vi "UI_sendComplexMessage.vi"(5 "Notif T/O":i32=250, 6 "notifier":refnum<notifier>, 7 "Wait for Response":bool, 8 "error in (no error)":errorcluster, 9 "Payload":variant, 10 "Command":string, 11 "Queue Bus":T1) -> (0 "error out":errorcluster, 1 "payload":variant, 3 "Queue Bus OUT":T1)   [LabVIEW 2020]
uses:
  Typedefs/queueBus.ctl
  Typedefs/communicationData.ctl
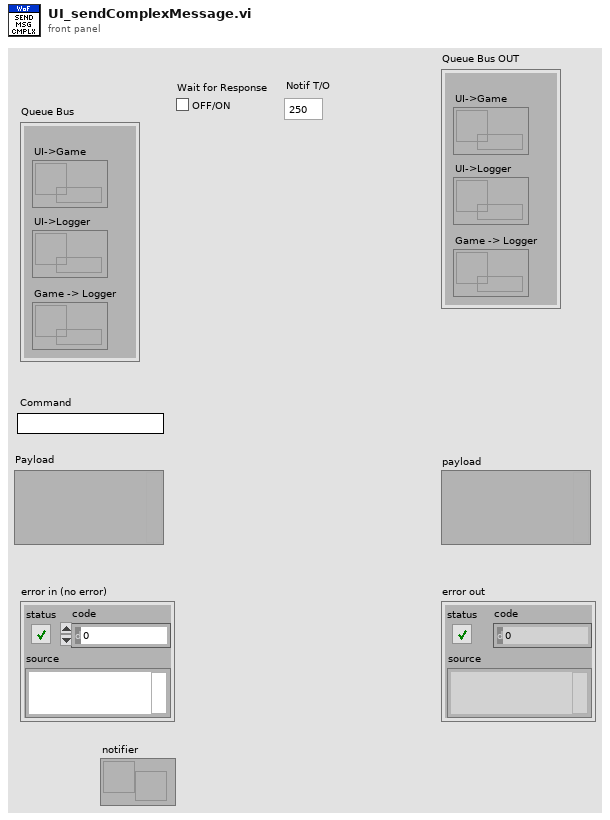
[diagram p1: front panel]
types:
  T1 = typedef "queueBus.ctl" = cluster{"UI->Game":refnum<queue>, "UI->Logger":refnum<queue>, "Game -> Logger":refnum<queue>}
  T2 = typedef "communicationData.ctl" = cluster{"command":string, "payload":variant, "response":variant}
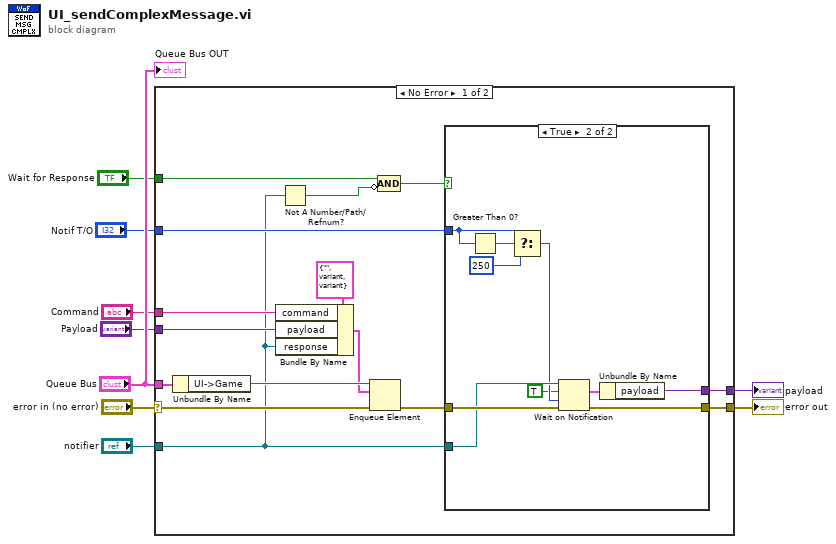
[diagram p0: block diagram]
diagram:
  n1 = case shown="No Error" "error in (no error)" {
    selector: "error in (no error)" -> [w22 w36]
    tunnel: [w15 w36] -> w7
    tunnel: "notifier" -> [w12 _]
    tunnel: "Queue Bus" -> [w24 _]
    tunnel: "Payload" -> [w19 _]
    tunnel: "Command" -> [w20 _]
    tunnel: "Wait for Response" -> [w17 _]
    tunnel: "Notif T/O" -> [w14 _]
    tunnel: [w13 _] -> w1
    frame No Error {
      n2 = Unbundle By Name(w24) -> ("UI->Game"=w23:refnum<queue>)
      n3 = Bundle By Name(cluster=T2 {"command"="", "payload"=variant, "response"=variant} ("communication"), "command"=w20, "payload"=w19, "response"=w12) -> (w18:T2)
      n4 = Not A Number/Path/Refnum?(number/path/refnum=w12) -> (NaN/Path/Refnum?=w10:bool)
      n5 = Enqueue Element(queue=w23, element=w18, error in (no error)=w22) -> (error out=w16:errorcluster)  [unwired: 1 in, 2 out]
      n6 = Compound Arithmetic op=AND(w17, invert w10) -> (w11:bool)
      n7 = case shown="True" w11 {
        tunnel: w16 -> [w25 w35]
        tunnel: [w25 w34] -> w15
        tunnel: w12 -> [_ w33]
        tunnel: w14 -> [_ w31]
        tunnel: [_ w26] -> w13
        frame False {
        }
        frame True {
          n8 = Greater Than 0?(x=w31) -> (x > 0?=w32:bool)
          n9 = Select(t=w31, s=w32, f=250) -> (s? t:f=w29:i32)
          n10 = Wait on Notification(notifier=w33, ignore previous (F)=TRUE, timeout in ms (-1)=w29, error in (no error)=w35) -> (notification=w27:T2, error out=w34:errorcluster)  [unwired: 2 out]
          n11 = Unbundle By Name(w27) -> ("payload"=w26:variant)
        }
      }
    }
    frame Error {
    }
  }
  "error out" <- w7
  "payload" <- w1
  "Queue Bus OUT" <- "Queue Bus"
